vi "testPM100.vi"() -> ()   [LabVIEW 2009, in "run.lvlib"]
uses:
  run.lvlib
panel:
  out "read buffer":string
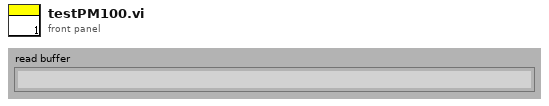
[diagram p1: front panel]
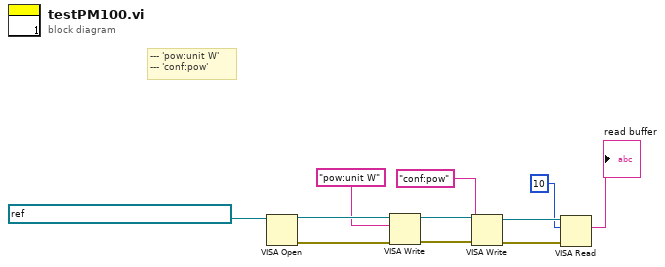
[diagram p0: block diagram]
diagram:
  # "--- 'pow:unit W'\n--- 'conf:pow'"
  n1 = VISA Open(VISA resource name=refnum<visa-resource-name> "pm100d") -> (VISA resource name=w10:refnum<visa-resource-name>, error out=w6:errorcluster)  [unwired: 4 in]
  n2 = VISA Write(VISA resource name=w10, write buffer="pow:unit W", error in (no error)=w6) -> (VISA resource name out=w8:refnum<visa-resource-name>, error out=w5:errorcluster)  [unwired: 1 out]
  n3 = VISA Write(VISA resource name=w8, write buffer="conf:pow", error in (no error)=w5) -> (VISA resource name out=w3:refnum<visa-resource-name>, error out=w4:errorcluster)  [unwired: 1 out]
  n4 = VISA Read(VISA resource name=w3, byte count=10, error in (no error)=w4) -> (read buffer=→"read buffer":string)  [unwired: 3 out]
